vi "Get Data.vi"(8 "error in":errorcluster, 11 "Test Device in":refnum<class "Test Device.lvclass">) -> (0 "error out":errorcluster, 2 "DataOut":refnum<class "Data.lvclass">, 3 "Test Device out":refnum<class "Test Device.lvclass">)   [LabVIEW 2014, in "Test Device.lvclass"]
uses:
  Test Device.lvclass
  reusable/Data/Data.lvclass
  Configurable Device.lvclass/Configurable Device.ctl
  Test Device.lvclass/Test Device.ctl
  reusable/Data/Data.lvclass/Data.ctl
  Read ID.vi
  reusable/Data/Write Data ID.vi
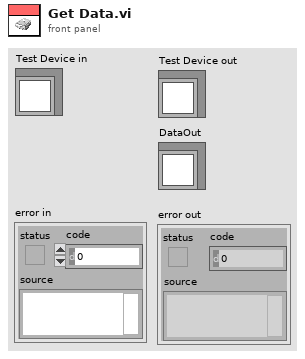
[diagram p1: front panel]
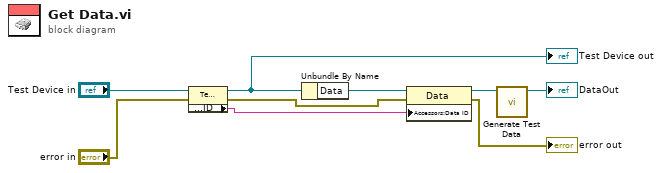
[diagram p0: block diagram]
diagram:
  n1 = property class="Test Device"(reference="Test Device in", error in="error in") -> (reference out=w1:refnum<class "Test Device.lvclass">, error out=w3:errorcluster, "Accessors:ID"=w6:string)
  "Test Device out" <- w1
  n2 = Unbundle By Name(w1) -> ("Data"=w7:refnum<class "Data.lvclass">)
  n3 = property class="Data"(reference=w7, error in=w3, "Accessors:Data ID"=w6) -> (reference out=w5:refnum<class "Data.lvclass">, error out=→"error out":errorcluster)
  n4 = call-dynamic "Generate Test Data.vi"("Data in"=w5) -> ("Data out"=→"DataOut":refnum<class "Data.lvclass">)  [unwired: 10 in]
